vi "量程参数复合参数写入.vi"(11 "备用系数":T1) -> ()   [LabVIEW 2016, in "斯坦道总磷.lvlib"]
uses:
  <vilib>/Utility/miscctls.llb/LVPointTypeDef.ctl
panel:
  in  "参数下拉列表":enum16{"总磷", "总氮"}(ring)
  in  "取消":bool
  in  "确认":bool
  # "请选择要写入的参数"
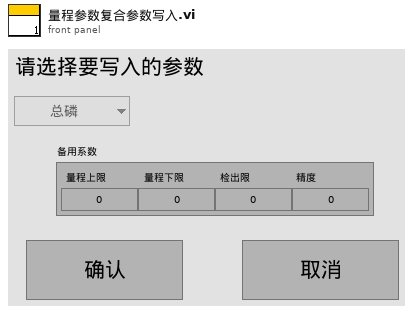
[diagram p1: front panel]
types:
  T1 = cluster{"量程上限":dbl, "量程下限":dbl, "检出限":dbl, "精度":dbl}
  T2 = typedef "LVPointTypeDef.ctl" = cluster{"Horizontal":i16, "Vertical":i16}
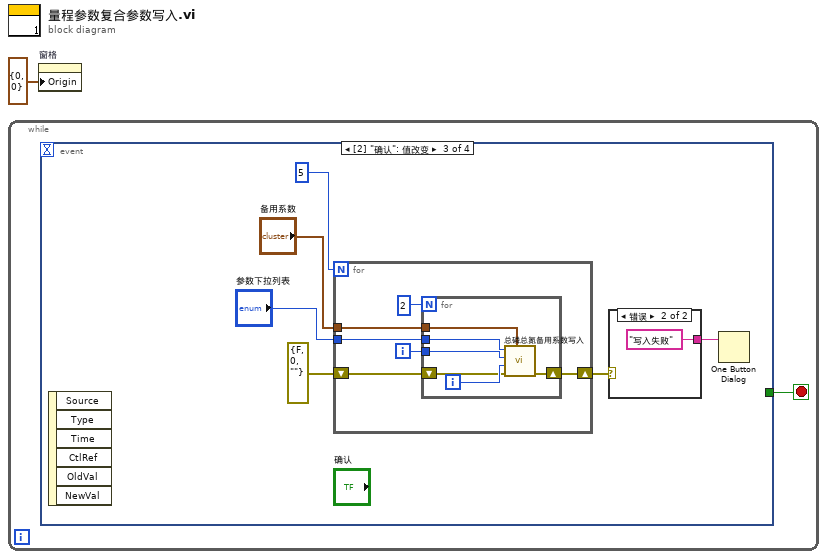
[diagram p0: block diagram]
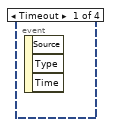
[diagram p2: hidden frame]
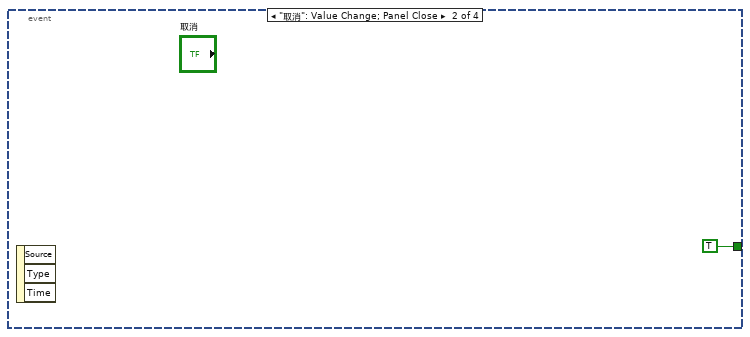
[diagram p3: hidden frame]
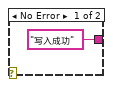
[diagram p4: hidden frame]
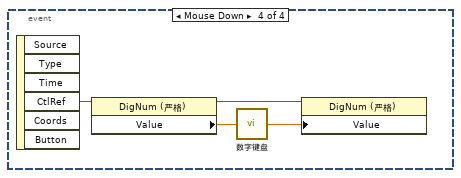
[diagram p5: hidden frame]
diagram:
  n1 = while {
    stop <- w2 stop-if-true
    n2 = event shown="[2] \"确认\": 值改变" {
      selector: _ -> [_ _ _ _]
      dyn-events: _ -> [_ _ _ _]
      timeout: _ -> [_ _ _ _]
      tunnel: [_ TRUE _ _] -> w2
      event Timeout {
        n3 = event-data() -> ()  [unwired: 1 in, 3 out]
      }
      event "取消": Value Change; Panel Close {
        n4 = event-data() -> ()  [unwired: 1 in, 3 out]
      }
      event "确认": Value Change {
        n5 = event-data() -> ()  [unwired: 1 in, 6 out]
        n6 = for {
          N: 5 -> [_]
          tunnel: "备用系数" -> [w17]
          tunnel: "参数下拉列表" -> [w16]
          shift-right: [w13] -> w5
          shift-left: errorcluster {"status"=FALSE, "code"=0, "source"=""} ("error out") -> [w12]
          i -> [w15]
          n7 = for {
            N: 2 -> [_]
            tunnel: w17 -> [w23]
            tunnel: w16 -> [w22]
            tunnel: w15 -> [w21]
            shift-right: [w19] -> w13
            shift-left: w12 -> [w18]
            i -> [w20]
            n8 = call "总磷总氮备用系数写入.vi"("备用系数"=w23, "error in (no error)"=w18, "量程"=w20, "测量模式"=w21, "测量参数"=w22) -> ("error out"=w19:errorcluster)  [unwired: 6 in]
          }
        }
        n9 = case shown="错误" w5 {
          tunnel: ["写入成功" ("消息") "写入失败" ("消息")] -> w4
          frame No Error {
          }
          frame Error {
          }
        }
        n10 = One Button Dialog(message=w4) -> ()  [unwired: 1 in, 1 out]
      }
      event "备用系数.量程上限", "备用系数.量程下限", "备用系数.检出限", "备用系数.精度": Mouse Down {
        n11 = event-data() -> ("CtlRef"=w27:refnum<vi>)  [unwired: 1 in, 5 out]
        n12 = property class="DigNum (严格)"(reference=w27) -> (reference out=w24:refnum<vi>, "Value"=w26:dbl)  [unwired: 1 in, 1 out]
        n13 = call "数字键盘.vi"("OldNumber"=w26) -> ("NewNumber"=w25:dbl)
        n14 = property class="DigNum (严格)"(reference=w24, "Value"=w25) -> ()  [unwired: 1 in, 2 out]
      }
    }
  }
  n15 = property on="窗格" class="Pane"("Origin"=T2 {"Horizontal"=0, "Vertical"=0} ("原点")) -> ()  [unwired: 2 in, 2 out]
